vi "Active object Event_Create.vi"(0 "reference in":refnum<class "Active object Event.lvclass">, 5 "error in (no error)":errorcluster) -> (14 "reference out":refnum<class "Active object Event.lvclass">, 19 "error out":errorcluster)   [LabVIEW 2019, in "Active object Event.lvclass"]
uses:
  Active object Event.lvclass
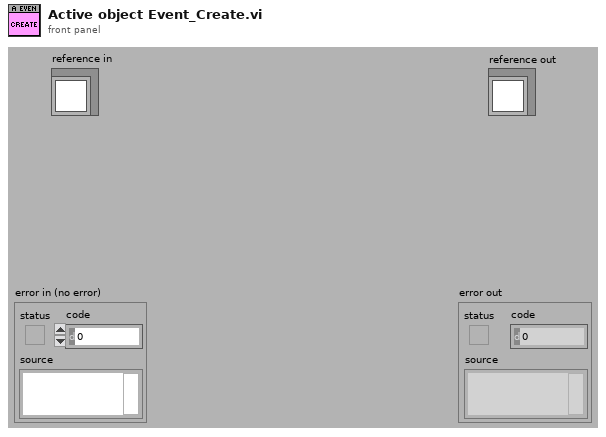
[diagram p1: front panel]
types:
  T1 = typedef "G4BaseTemplate_Simple_6x8x6.lvclass/ObjectAttributes.ctl" = cluster{"Attribute1":dbl}
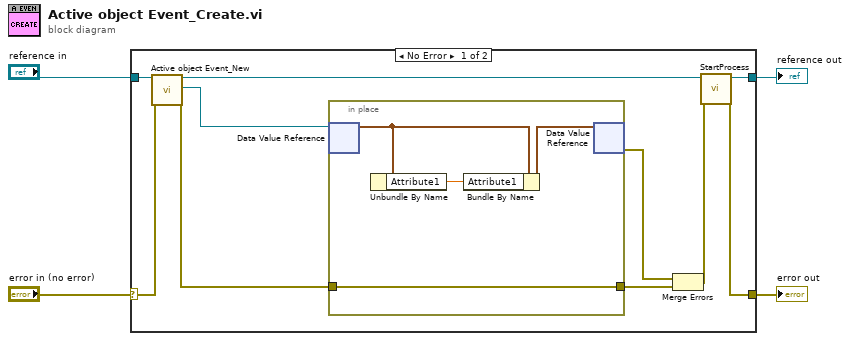
[diagram p0: block diagram]
diagram:
  n1 = case shown="No Error" "error in (no error)" {
    selector: "error in (no error)" -> [w13 w20]
    tunnel: [w5 w20] -> w3
    tunnel: "reference in" -> [w14 w19]
    tunnel: [w7 w19] -> w1
    frame No Error {
      n2 = call "Active object Event_New.vi"("reference in"=w14, "error in (no error)"=w13) -> ("reference out"=w8:refnum<class "Active object Event.lvclass">, "DVRRefOut"=w11:refnum<data-value>, "error out"=w10:errorcluster)  [unwired: 14 in, 1 out]
      n3 = in-place {
        in-place-border: w10 -> [w15]
        in-place-border: [w15] -> w9
        n4 = in-place-dvr #1(w11) -> (w17:T1)  [unwired: 1 out]
        n5 = Unbundle By Name(w17) -> ("Attribute1"=w16:dbl)
        n6 = Bundle By Name(cluster=w17, "Attribute1"=w16) -> (w18:T1)
        n7 = in-place-dvr #1(w18) -> (w12:errorcluster)  [unwired: 1 out]
      }
      n8 = Merge Errors(w12, w9) -> (w6:errorcluster)
      n9 = call "StartProcess.vi"("reference in"=w8, "error in (no error)"=w6) -> ("reference out"=w7:refnum<class "Active object Event.lvclass">, "error out"=w5:errorcluster)  [unwired: 14 in, 2 out]
    }
    frame Error {
    }
  }
  "error out" <- w3
  "reference out" <- w1
